vi "零件加工.vi"(8 "error in (no error)":errorcluster caption="错误输入（无错误）", 11 "加工中心 输入":refnum<class "加工中心.lvclass"> caption="DNL_LabVIEW Object in") -> (0 "error out":errorcluster caption="错误输出", 3 "加工中心 输出":refnum<class "加工中心.lvclass"> caption="DNL_LabVIEW Object out")   [LabVIEW 2011, in "加工中心.lvclass"]
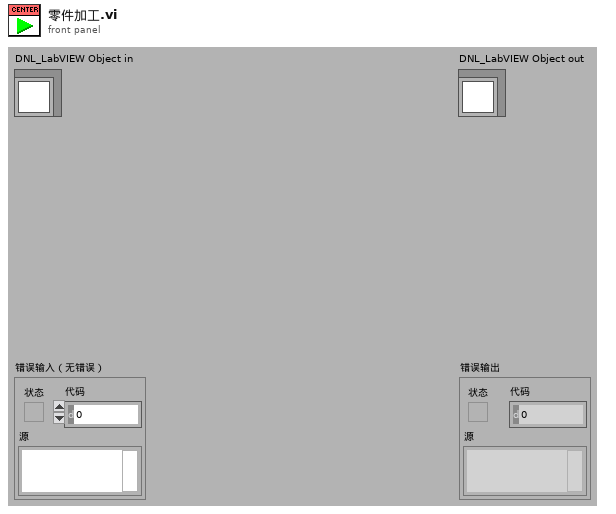
[diagram p1: front panel]
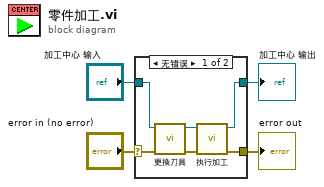
[diagram p0: block diagram]
diagram:
  n1 = case shown="无错误" "error in (no error)" {
    selector: "error in (no error)" -> [w7 w12]
    tunnel: [w5 w12] -> w3
    tunnel: [w8 w11] -> w1
    tunnel: "加工中心 输入" -> [w10 w11]
    frame No Error {
      n2 = call "更换刀具.vi"("error in (no error)"=w7, "加工中心 输入"=w10) -> ("error out"=w6:errorcluster, "加工中心 输出"=w9:refnum<class "加工中心.lvclass">)  [unwired: 8 in]
      n3 = call "执行加工.vi"("error in (no error)"=w6, "加工中心 输入"=w9) -> ("error out"=w5:errorcluster, "加工中心 输出"=w8:refnum<class "加工中心.lvclass">)  [unwired: 8 in]
    }
    frame Error {
    }
  }
  "error out" <- w3
  "加工中心 输出" <- w1
